vi "PipBoy_CheckPipConnection.vi"(8 "error in (no error)":errorcluster, 11 "VISAPic32":refnum<visa-resource-name>) -> (0 "error out":errorcluster, 2 "Error ?":bool)   [LabVIEW 2014]
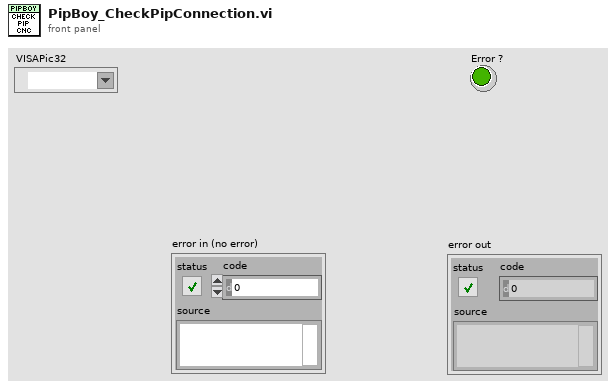
[diagram p1: front panel]
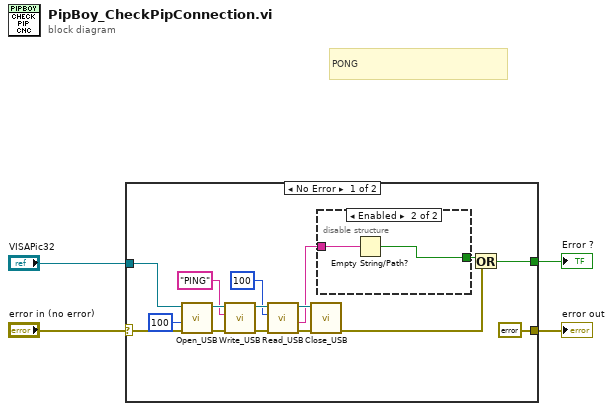
[diagram p0: block diagram]
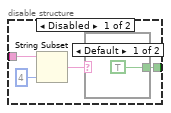
[diagram p2: hidden frame]
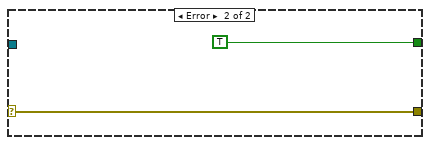
[diagram p4: hidden frame]
diagram:
  # "PONG"
  n1 = case shown="No Error" "error in (no error)" {
    selector: "error in (no error)" -> [w10 w29]
    tunnel: [errorcluster {"status"=FALSE, "code"=0, "source"=""} ("error IO") w29] -> w3
    tunnel: [w11 TRUE] -> w2
    tunnel: "VISAPic32" -> [w8 _]
    frame No Error {
      n2 = call "Open_USB.vi"("entrée d'erreur"=w10, "Timeout (100)"=u32 100 ("Timeout (0)"), "Nom de ressource VISA"=w8) -> ("error out"=w16:errorcluster, "Nom de ressource VISA ouverte"=w20:refnum<visa-resource-name>)  [unwired: 7 in]
      n3 = call "Write_USB.vi"("entrée d'erreur"=w16, "buffer d'écriture"="PING", "Nom de ressource VISA"=w20) -> ("sortie d'erreur"=w15:errorcluster, "Nom de ressource VISA en sortie"=w19:refnum<visa-resource-name>)  [unwired: 7 in]
      n4 = call "Read_USB.vi"("entrée d'erreur"=w15, "timeout (0)"=u32 100, "Nom de ressource VISA"=w19) -> ("sortie d'erreur"=w14:errorcluster, "chaîne en sortie"=w7:string, "Nom de ressource VISA en sortie"=w17:refnum<visa-resource-name>)  [unwired: 6 in]
      n5 = call "Close_USB.vi"("entrée d'erreur"=w14, "Nom de ressource VISA"=w17) -> ("sortie d'erreur"=w12:errorcluster)  [unwired: 9 in]
      n6 = disable-structure shown="Enabled" {
        disable-tunnel: [w24 w26] -> w13
        disable-tunnel: w7 -> [w22 w27]
        frame Disabled {
          n7 = String Subset(string=w22, length (rest)=4 ("length (rest)")) -> (substring=w21:string)  [unwired: 1 in]
          n8 = case shown="Default" w21 {
            tunnel: [TRUE _] -> w24
            frame Default {
            }
            frame "PONG" {
            }
          }
        }
        frame Enabled {
          n9 = Empty String/Path?(string/path=w27) -> (empty?=w26:bool)
        }
      }
      n10 = Or(x=w13, y=w12) -> (x .or. y?=w11:bool)
    }
    frame Error {
    }
  }
  "error out" <- w3
  "Error ?" <- w2
